vi "test Diff Configuration (No Change).vi"(8 "error in":errorcluster, 11 "TestCase in":refnum<class "Refresh.lvclass">) -> (0 "error out":errorcluster, 3 "TestCase out":refnum<class "Refresh.lvclass">)   [LabVIEW 2020, in "Refresh.lvclass"]
uses:
  Refresh.lvclass
  Shared/BIU Configuration.ctl
  Shared/Address.ctl
  Shared/Major Frame Definition.ctl
  Shared/Minor Frame Definition.ctl
  Shared/Acyclic Frame Definition.ctl
  Shared/Message Definition.ctl
  Shared/Message Type.ctl
  Shared/Terminal Endpoint.ctl
  Shared/Parameter Definition.ctl
  System Explorer/Implementation/System Explorer/Refresh/Change Type.ctl
  <vilib>/addons/_JKI Toolkits/VI Tester/TestCase.llb/TestCase.lvclass
  System Explorer/Implementation/System Explorer/Refresh/Refresh.lvlib
  C:/Program Files (x86)/National Instruments/LabVIEW 2020/vi.lib/addons/_JKI Toolkits/VI Tester/TestCase.llb/TestCase.lvclass
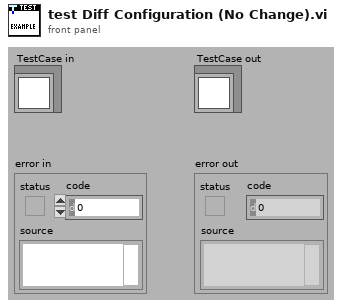
[diagram p1: front panel]
types:
  T1 = typedef "BIU Configuration.ctl" = cluster{"HW channel":u16, "terminal addresses":T2[], "terminal names":string[], "major frames":T3[], "minor frames":T4[], "acyclic frames":T5[], "messages":T6[], "minor frame period (us)":i32, "starting buffer index":u16}
  T2 = typedef "Address.ctl" = u16
  T3 = typedef "Major Frame Definition.ctl" = cluster{"name":string, "minor frames":string[]}
  T4 = typedef "Minor Frame Definition.ctl" = cluster{"name":string, "messages":string[]}
  T5 = typedef "Acyclic Frame Definition.ctl" = cluster{"name":string, "messages":string[]}
  T6 = typedef "Message Definition.ctl" = cluster{"name":string, "message type":T7, "endpoint Tx":T8, "endpoint Rx":T8, "create timestamp channel":bool, "mode code":u16, "number of words":u16, "parameters":cluster{"name":string, "default value":dbl, "unit":string, "parameter definition":T9}[]}
  T7 = typedef "Message Type.ctl" = string
  T8 = typedef "Terminal Endpoint.ctl" = cluster{"terminal address":T2, "subaddress":T2}
  T9 = typedef "Parameter Definition.ctl" = cluster{"start index":i32, "size (bits)":i32, "encoding":enum16{"BNR", "BCD", "Discrete"}, "signed":bool, "multiplier":dbl, "offset":dbl}
  T10 = typedef "AIM MIL-STD-1553 System Explorer.lvlib/Implementation.lvlib/Refresh.lvlib/Change Type.ctl" = enum16{"No change", "Modify", "Add", "Remove"}
  T11 = typedef "AIM MIL-STD-1553 System Explorer.lvlib/Implementation.lvlib/Refresh.lvlib/MCL Row.ctl" = cluster{"change type":T10, "item symbol":T12, "item names":string[]}
  T12 = typedef "AIM MIL-STD-1553 System Explorer.lvlib/Implementation.lvlib/Refresh.lvlib/Symbols.ctl" = enum16{"Blank", "MIL-STD-1553", "Port", "Remote Terminal", "Subaddress", "Bus Controller", "Frame", "Mode Code", "Message", "Parameter", "Item"}
  T13 = cluster{"name":string, "default value":dbl, "unit":string, "parameter definition":T9}[]
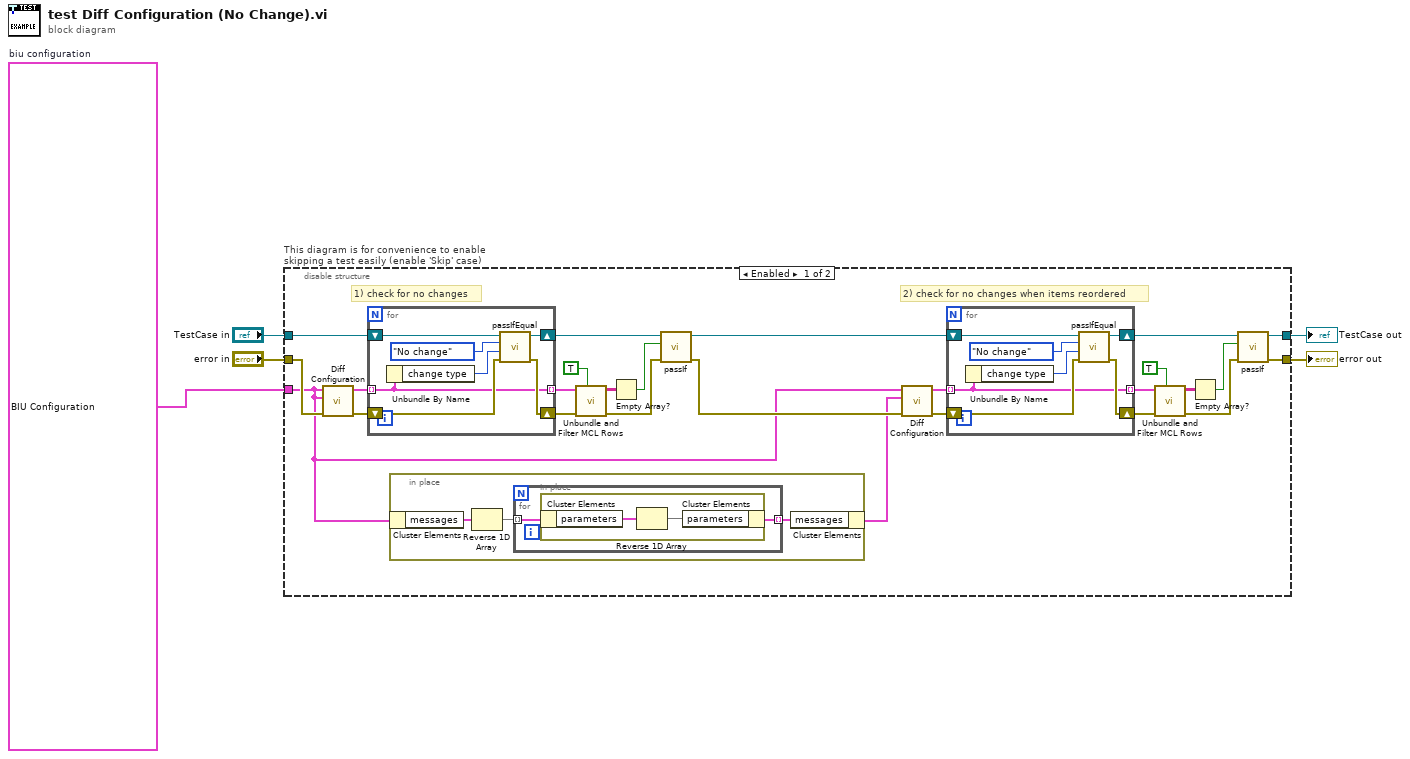
[diagram p0: block diagram]
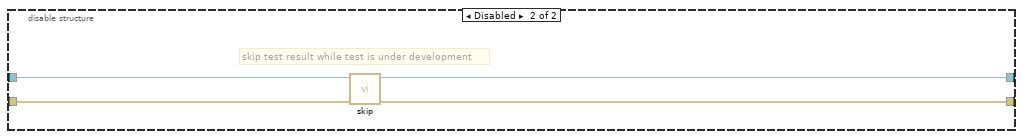
[diagram p2: hidden frame]
diagram:
  w1 = T1 {"HW channel"=0, "terminal addresses"=[0, 1, 2], "terminal names"=[], "major frames"=[{"name"="A1", "minor frames"=[]}], "minor frames"=[{"name"="A2", "messages"=[]}, {"name"="A6", "messages"=[]}, {"name"="A7", "messages"=[]}], "acyclic frames"=[{"name"="A3", "messages"=[]}, {"name"="A6", "messages"=[]}], "messages"=[{"name"="Message 001", "message type"="BC to RT", "endpoint Tx"={"terminal address"=1, "subaddress"=1}, "endpoint Rx"={"terminal address"=0, "subaddress"=0}, "create timestamp channel"=TRUE, "mode code"=0, "number of words"=3, "parameters"=[{"name"="Word0", "default value"=1.0, "unit"="eu", "parameter definition"={"start index"=0, "size (bits)"=16, "encoding"=enum."BNR", "signed"=FALSE, "multiplier"=1.0, "offset"=0.0}}, {"name"="Word1", "default value"=1.0, "unit"="eu", "parameter definition"={"start index"=16, "size (bits)"=16, "encoding"=enum."BNR", "signed"=TRUE, "multiplier"=1.0, "offset"=0.0}}, {"name"="Word2", "default value"=1.0, "unit"="eu", "parameter definition"={"start index"=32, "size (bits)"=16, "encoding"=enum."BNR", "signed"=TRUE, "multiplier"=1.0, "offset"=0.0}}]}], "minor frame period (us)"=0, "starting buffer index"=0}  # biu configuration
  n1 = disable-structure "This diagram is for convenience to enable skipping a test easily (enable 'Skip' case)" shown="Enabled" {
    disable-tunnel: "TestCase in" -> [w30 w56]
    disable-tunnel: [w6 w54] -> w2
    disable-tunnel: [w7 w55] -> w4
    disable-tunnel: "error in" -> [w31 w53]
    disable-tunnel: w1 -> [w9 _]
    frame Enabled {
      # "2) check for no changes when items reordered"
      # "1) check for no changes"
      n2 = call "Diff Configuration.vi"("error in"=w31, "configuration new"=w9, "configuration old"=w9) -> ("error out"=w25:errorcluster, "configuration diff"=w24:T11[])  [unwired: 7 in]
      n3 = for {
        shift-right: [w51] -> w26
        shift-left: w30 -> [w52]
        shift-right: [w47] -> w22
        shift-left: w25 -> [w48]
        tunnel: w24 -> [w46] mode=indexing
        tunnel: [w46] -> w23 mode=indexing
        n4 = Unbundle By Name(w46) -> ("change type"=w49:T10)
        n5 = call-dynamic "passIfEqual.vi"("error in (no error)"=w48, "y"=w49, "x"=Change_Type."No change" ("change type"), "TestCase in"=w52) -> ("error out"=w47:errorcluster, "TestCase out"=w51:refnum<class "Refresh.lvclass">)  [unwired: 6 in]
      }
      n6 = in-place {
        n7 = in-place-cluster #1(w9) -> ("messages"=w33:T6[])
        n8 = Reverse 1D Array(array=w33) -> (reversed array=w34:T6[])
        n9 = for {
          tunnel: w34 -> [w36] mode=indexing
          tunnel: [w35] -> w32 mode=indexing
          n10 = in-place {
            n11 = in-place-cluster #2(w36) -> ("parameters"=w38:T13)
            n12 = Reverse 1D Array(array=w38) -> (reversed array=w37:T13)
            n13 = in-place-cluster #2("parameters"=w37) -> (w35:T6)
          }
        }
        n14 = in-place-cluster #1("messages"=w32) -> (w8:T1)
      }
      n15 = call "Unbundle and Filter MCL Rows.vi"("filter changed items"=TRUE, "error in"=w22, "refresh items"=w23) -> ("error out"=w21:errorcluster, "item names"=w28:string[][])  [unwired: 5 in, 2 out]
      n16 = Empty Array?(array=w28) -> (empty?=w27:bool)
      n17 = call-dynamic "passIf.vi"("error in (no error)"=w21, "pass"=w27, "TestCase in"=w26) -> ("error out"=w10:errorcluster, "TestCase out"=w11:refnum<class "Refresh.lvclass">)  [unwired: 7 in]
      n18 = call "Diff Configuration.vi"("error in"=w10, "configuration new"=w8, "configuration old"=w9) -> ("error out"=w16:errorcluster, "configuration diff"=w17:T11[])  [unwired: 7 in]
      n19 = for {
        shift-right: [w44] -> w15
        shift-left: w11 -> [w45]
        shift-right: [w40] -> w19
        shift-left: w16 -> [w41]
        tunnel: w17 -> [w39] mode=indexing
        tunnel: [w39] -> w18 mode=indexing
        n20 = Unbundle By Name(w39) -> ("change type"=w42:T10)
        n21 = call-dynamic "passIfEqual.vi"("error in (no error)"=w41, "y"=w42, "x"=Change_Type."No change" ("change type"), "TestCase in"=w45) -> ("error out"=w40:errorcluster, "TestCase out"=w44:refnum<class "Refresh.lvclass">)  [unwired: 6 in]
      }
      n22 = call "Unbundle and Filter MCL Rows.vi"("filter changed items"=TRUE, "error in"=w19, "refresh items"=w18) -> ("error out"=w20:errorcluster, "item names"=w13:string[][])  [unwired: 5 in, 2 out]
      n23 = Empty Array?(array=w13) -> (empty?=w14:bool)
      n24 = call-dynamic "passIf.vi"("error in (no error)"=w20, "pass"=w14, "TestCase in"=w15) -> ("error out"=w7:errorcluster, "TestCase out"=w6:refnum<class "Refresh.lvclass">)  [unwired: 7 in]
    }
    frame Disabled {
      # "skip test result while test is under development"
      n25 = call <vilib>:"skip.vi"("error in (no error)"=w53, "TestCase in"=w56) -> ("error out"=w55:errorcluster, "TestCase out"=w54:refnum<class "Refresh.lvclass">)  [unwired: 8 in]
    }
  }
  "error out" <- w4
  "TestCase out" <- w2
